vi "check_is_moving.vi"(8 "error in (no error)":errorcluster, 11 "dummyStage in":refnum<class "dummyStage.lvclass">) -> (0 "error out":errorcluster, 2 "number":dbl, 3 "dummyStage out":refnum<class "dummyStage.lvclass">)   [LabVIEW 2019, in "dummyStage.lvlib" / "dummyStage.lvclass"]
uses:
  dummyStage.lvclass
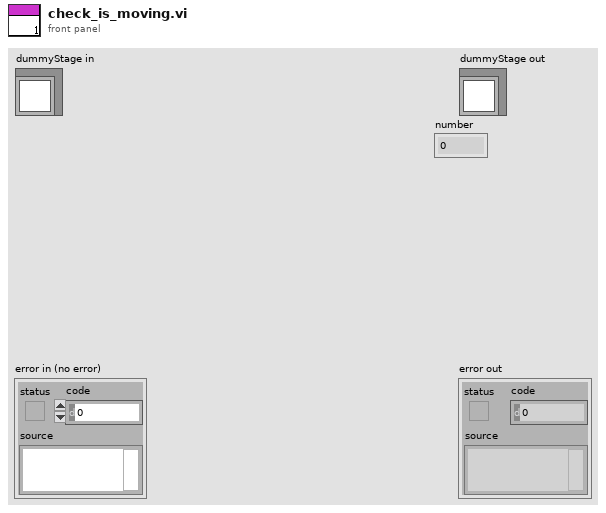
[diagram p1: front panel]
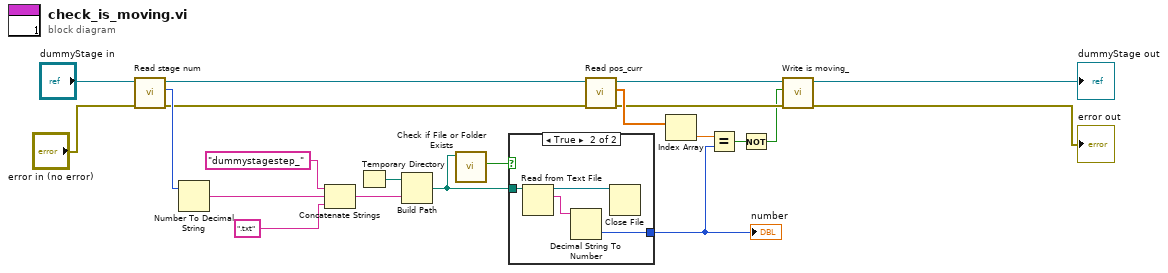
[diagram p0: block diagram]
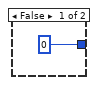
[diagram p2: hidden frame]
diagram:
  n1 = call-dynamic "Read stage num.vi"("error in (no error)"="error in (no error)", "_stage in"="dummyStage in") -> ("error out"=w14:errorcluster, "stage num"=w19:u8, "_stage out"=w15:refnum<class "dummyStage.lvclass">)  [unwired: 7 in]
  n2 = Number To Decimal String(number=w19) -> (decimal integer string=w18:string)  [unwired: 1 in]
  n3 = Concatenate Strings("dummystagestep_", w18, ".txt") -> (w16:string)
  n4 = Temporary Directory() -> (w3:path)
  n5 = Build Path(base path=w3, name or relative path=w16) -> (appended path=w2:path)
  n6 = call <vilib>:"Check if File or Folder Exists.vi"("path"=w2) -> ("file or folder exists?"=w1:bool)  [unwired: 8 in, 2 out]
  n7 = case shown="True" w1 {
    tunnel: [0 w24] -> w13
    tunnel: w2 -> [_ w23]
    frame False {
    }
    frame True {
      n8 = Read from Text File(file (use dialog)=w23) -> (refnum out=w25:refnum<file>, text=w26:string)  [unwired: 3 in, 2 out]
      n9 = Decimal String To Number(string=w26) -> (number=w24:i32)  [unwired: 2 in, 1 out]
      n10 = Close File(refnum=w25) -> ()  [unwired: 1 in, 2 out]
    }
  }
  "number" <- w13
  n11 = call-dynamic "Read pos_curr.vi"("error in (no error)"=w14, "_stage in"=w15) -> ("error out"=w9:errorcluster, "readback position"=w12:dbl[], "_stage out"=w10:refnum<class "dummyStage.lvclass">)  [unwired: 7 in]
  n12 = Index Array(array=w12) -> (element=w11:dbl)  [unwired: 1 in]
  n13 = Equal?(x=w11, y=w13) -> (x = y?=w6:bool)
  n14 = Not(x=w6) -> (.not. x?=w5:bool)
  n15 = call-dynamic "Write is moving_.vi"("error in (no error)"=w9, "is moving?"=w5, "_stage in"=w10) -> ("error out"=→"error out":errorcluster, "_stage out"=→"dummyStage out":refnum<class "dummyStage.lvclass">)  [unwired: 7 in]
